vi "Actor Core.vi"(8 "error in":errorcluster, 11 "Monitor in":refnum<class "Classic Monitor.lvclass">) -> (0 "error out":errorcluster, 3 "Actor out":refnum<class "Actor.lvclass">)   [LabVIEW 2023, in "Monitored Actor.lvlib" / "Classic Monitor.lvclass"]
doc: "(<B>Filename</B>: Actor Framework.lvlib:Actor.lvclass:Actor Core.vi)\n\nReceives messages to the actor, reacts to them, and initiates any error handling that may shut the actor down.\n\nDescendant classes may override this VI to append parallel tasks for the actor to complete while it handles messages. Overrides use the Call Parent Method node."
uses:
  Classic Monitor.lvclass
  C:/Users/Public/Documents/Development/builds/Framework/Actor Framework.lvlibp/1abvi3w/vi.lib/ActorFramework/Actor/Actor.lvclass
  builds/Framework/Actor Framework.lvlibp/1abvi3w/vi.lib/ActorFramework/Actor/Actor.lvclass
  Monitor Data/Monitor Data.lvclass
  builds/Framework/Actor Framework.lvlibp/1abvi3w/vi.lib/ActorFramework/Message Enqueuer/Message Enqueuer.lvclass
  Classic Monitor.lvclass/Classic Monitor.ctl
  builds/Framework/Actor Framework.lvlibp/1abvi3w/vi.lib/ActorFramework/Time-Delayed Send Message/Time-Delay Override Options.ctl
  Orphan Detector/Orphan Detector/Orphan Detector.lvclass
  Actor Monitor/Actor Monitor Messages/Ping Actor Msg/Ping Actor Msg.lvclass
  C:/Users/Public/Documents/Development/builds/Framework/Actor Framework.lvlibp/1abvi3w/vi.lib/ActorFramework/Message/Message.lvclass
  Actor Monitor/Actor Monitor/Actor Monitor.lvclass
  Actor Monitor/Actor Monitor Messages/Manually Remove Actor Msg/Manually Remove Actor Msg.lvclass
  Monitor Messages/Log Messages Msg/Log Messages Msg.lvclass
  builds/Framework/Actor Framework.lvlibp/1abvi3w/vi.lib/ActorFramework/Stop Msg/Stop Msg.lvclass
  builds/Framework/Actor Framework.lvlibp
panel:
  in  "Monitored Actors":string[](tree)
  in  "Stop Actor":bool
  in  "Show Actor Core":bool
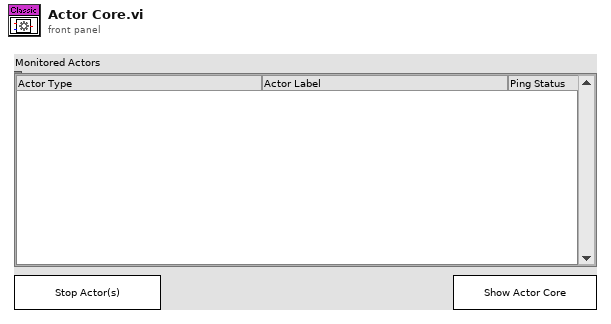
[diagram p1: front panel]
types:
  T1 = enum32{"Invalid", "Standard", "Closed", "Hidden", "Minimized", "Maximized"}
  T2 = cluster{"Monitor Data":refnum<class "Monitor Data.lvclass">, "Changed Actor Q":refnum<class "Message Enqueuer.lvclass">}
  T3 = cluster{"left":i16, "top":i16, "right":i16, "bottom":i16}
  T4 = typedef "Actor Framework.lvlibp/Time-Delay Override Options.ctl" = enum16{"Send next copy now", "Skip next scheduled copy", "Send next copy now and stop all further copies", "Stop all further copies"}
  T5 = enum8{"Enabled", "Disabled", "Disabled and Grayed Out"}
  T6 = typedef "LVRectTypeDef.ctl" = cluster{"Left":i16, "Top":i16, "Right":i16, "Bottom":i16}
  T7 = typedef "LVPoint32TypeDef.ctl" = cluster{"Horizontal":i32, "Vertical":i32}
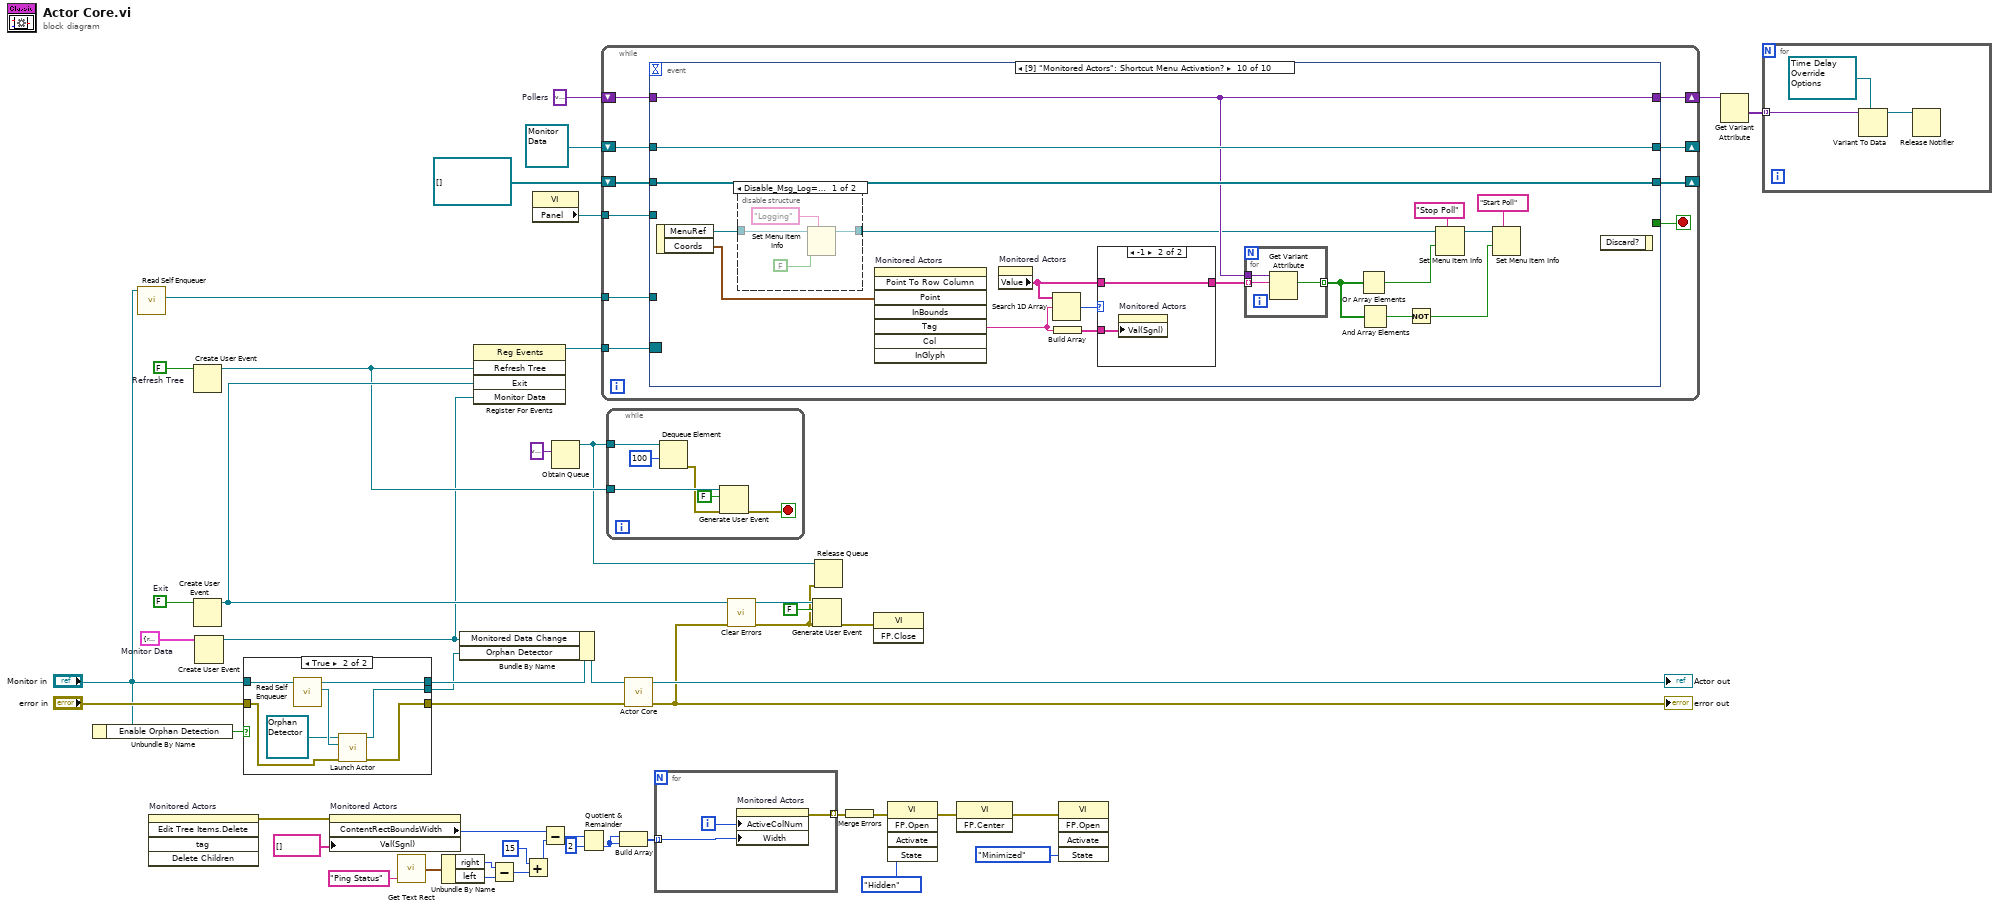
[diagram p0: block diagram]
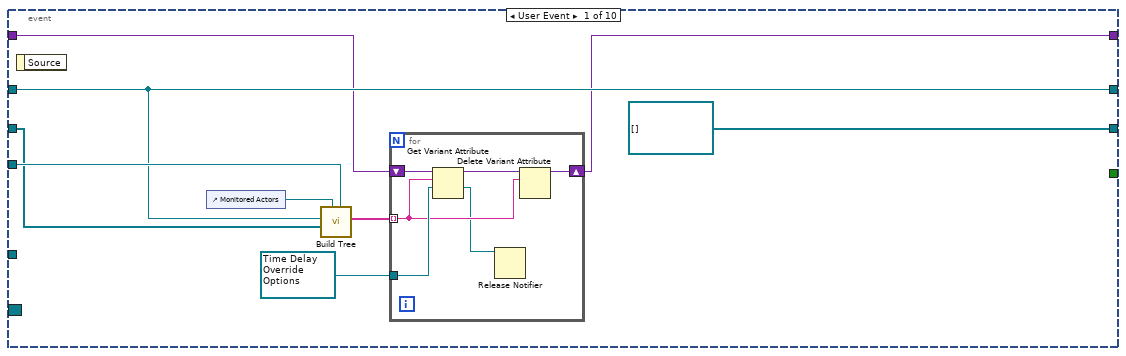
[diagram p3: hidden frame]
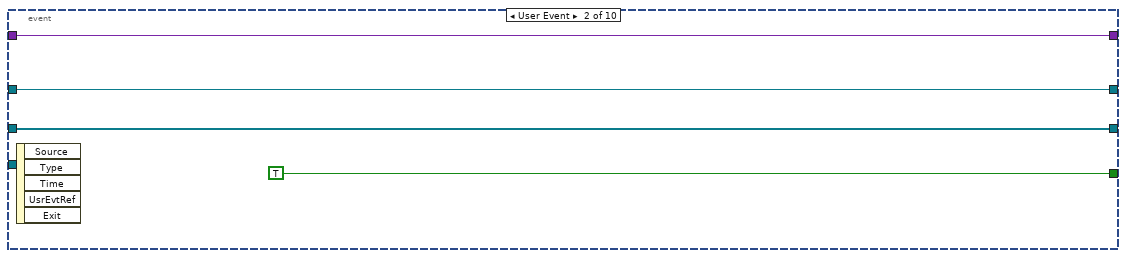
[diagram p4: hidden frame]
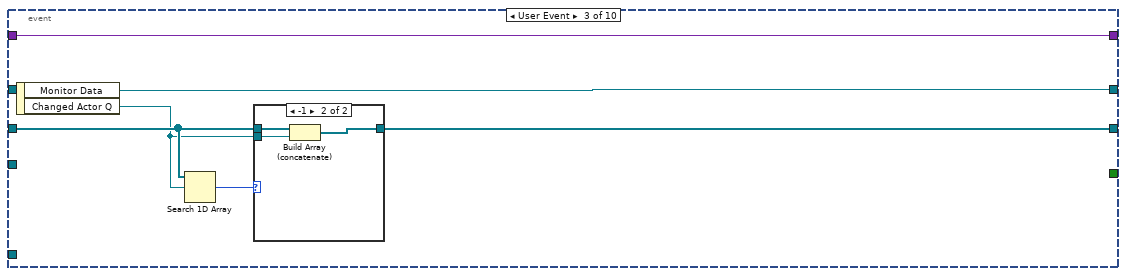
[diagram p5: hidden frame]
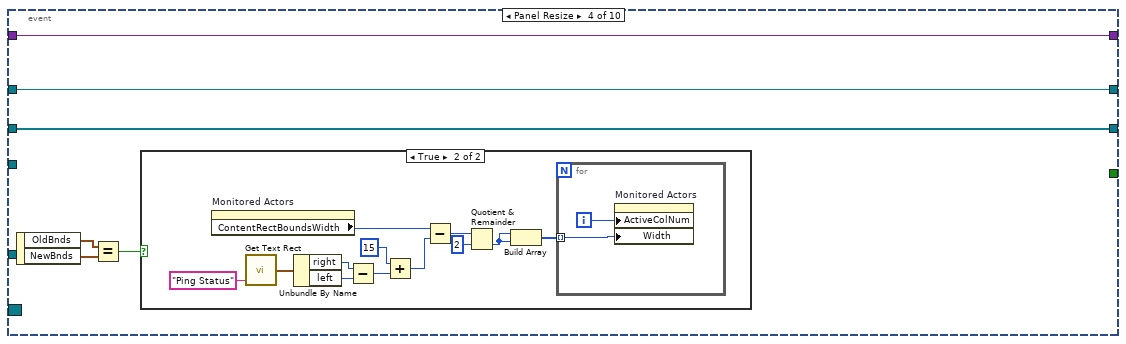
[diagram p7: hidden frame]
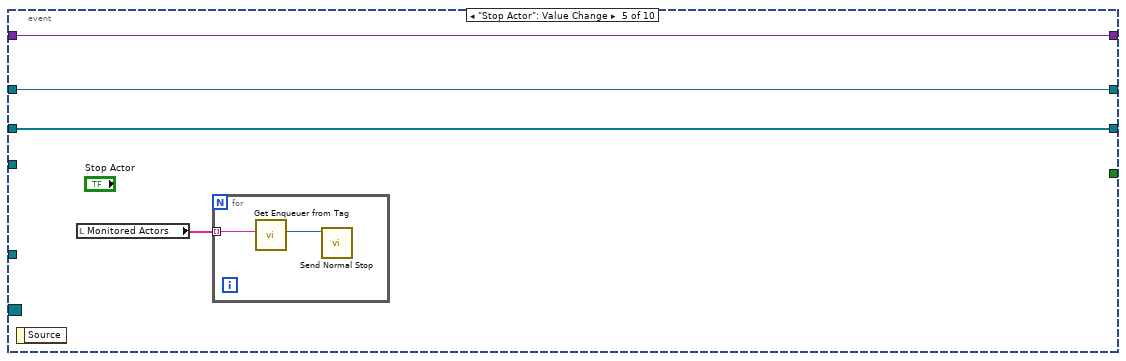
[diagram p9: hidden frame]
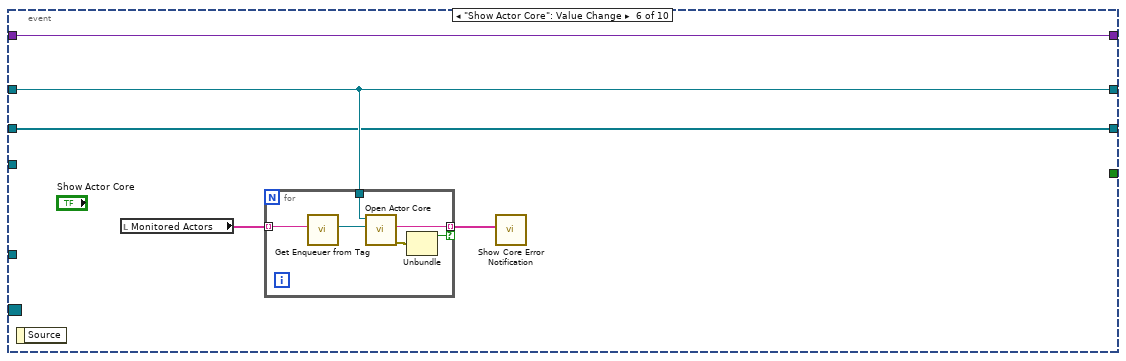
[diagram p10: hidden frame]
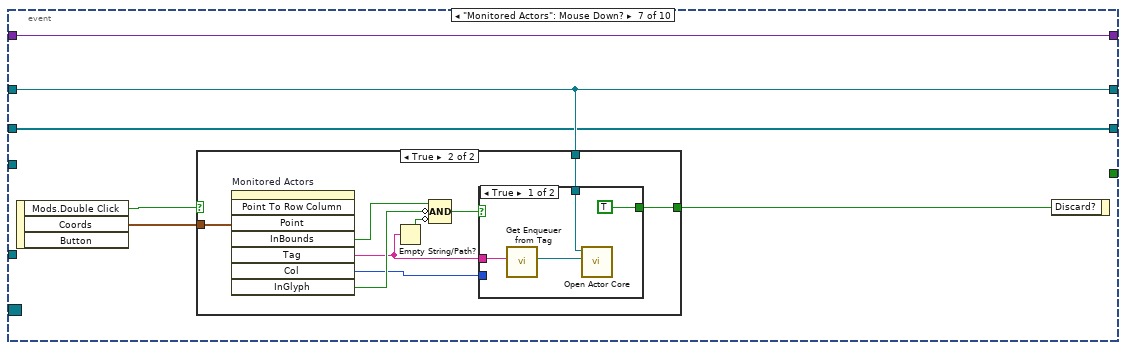
[diagram p11: hidden frame]
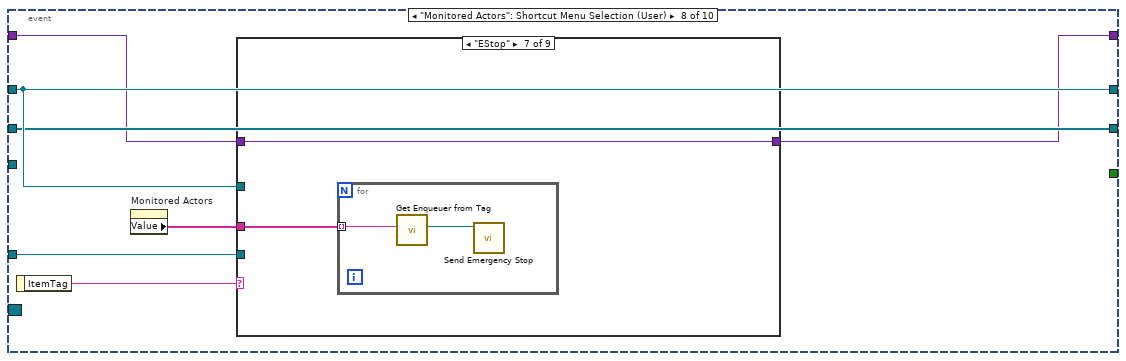
[diagram p14: hidden frame]
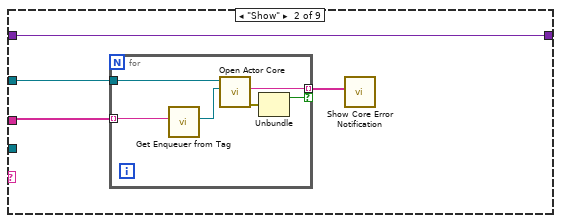
[diagram p16: hidden frame]
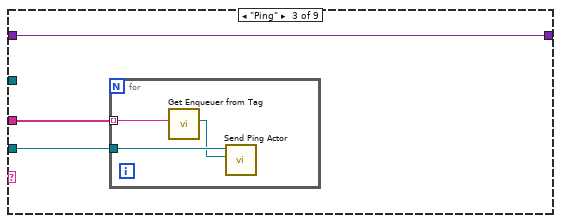
[diagram p17: hidden frame]
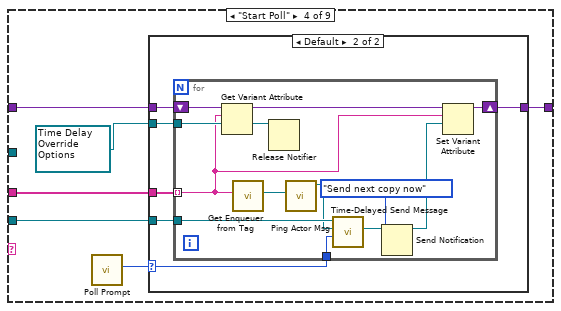
[diagram p18: hidden frame]
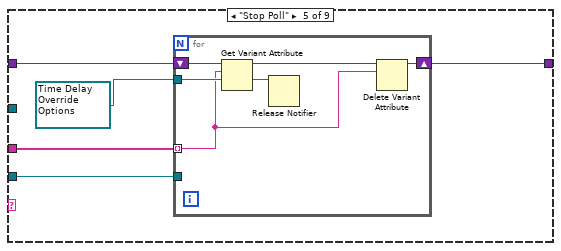
[diagram p20: hidden frame]
diagram:
  w5 = variant  # Pollers
  w15 = T2 {"Monitor Data"=refnum, "Changed Actor Q"=refnum}  # Monitor Data
  w20 = FALSE  # Refresh Tree
  w33 = FALSE  # Exit
  n1 = Unbundle By Name("Monitor in") -> ("Enable Orphan Detection"=w6:bool)
  n2 = call "Read Self Enqueuer.vi"("Actor"="Monitor in") -> ("Self Enqueuer"=w27:refnum<class "Message Enqueuer.lvclass">)  [unwired: 10 in]
  n3 = invoke on="Monitored Actors" class="Tree (strict)" method="Edit Tree Items.Delete"() -> (error out=w12:errorcluster)  [unwired: 5 in, 4 out]
  n4 = Create User Event(user event datatype=w20) -> (user event=w19:refnum<user-event>)  [unwired: 1 in, 1 out]
  n5 = Create User Event(user event datatype=w33) -> (user event=w32:refnum<user-event>)  [unwired: 1 in, 1 out]
  n6 = Create User Event(user event datatype=w15) -> (user event=w14:refnum<user-event>)  [unwired: 1 in, 1 out]
  n7 = case shown="True" w6 {
    tunnel: "error in" -> [w49 w52]
    tunnel: [w49 w51] -> w11
    tunnel: [w50 w55] -> w10
    tunnel: "Monitor in" -> [w50 w55]
    tunnel: [_ w53] -> w9
    frame False {
    }
    frame True {
      n8 = call "Read Self Enqueuer.vi"("Actor"=w55) -> ("Self Enqueuer"=w56:refnum<class "Message Enqueuer.lvclass">)  [unwired: 10 in]
      n9 = call "Launch Actor.vi"("error in (no error)"=w52, "Actor-to-Caller Enqueuer"=w56, "Actor"=refnum<class "Orphan Detector.lvclass"> refnum ("Classic Monitor.lvlib:Orphan Detector.lvclass")) -> ("error out"=w51:errorcluster, "Caller-To-Actor Enqueuer"=w53:refnum<class "Message Enqueuer.lvclass">)  [unwired: 7 in]
    }
  }
  n10 = property on="Monitored Actors" class="Tree (strict)"(error in=w12, "Val(Sgnl)"=string[] [] ("Value (Signaling)")) -> ("ContentRectBoundsWidth"=w46:i32)  [unwired: 1 in, 2 out]
  n11 = call <vilib>:"Get Text Rect.vi"("text"="Ping Status") -> ("rect"=w44:T3)  [unwired: 8 in]
  n12 = Unbundle By Name(w44) -> ("right"=w43:i16, "left"=w42:i16)
  n13 = Bundle By Name(cluster=w10, "Monitored Data Change"=w14, "Orphan Detector"=w9) -> (w30:refnum<class "Classic Monitor.lvclass">)
  n14 = register-events(w19, w32, w14) -> (reference out=w34:refnum<event-registration>)  [unwired: 2 in, 1 out]
  n15 = Subtract(x=w43, y=w42) -> (x-y=w41:i16)
  n16 = Add(x=i16 15, y=w41) -> (x+y=w38:i16)
  n17 = property class="VI"() -> ("Panel"=w28:refnum<vi>)  [unwired: 2 in, 2 out]
  n18 = Subtract(x=w46, y=w38) -> (x-y=w40:i32)
  n19 = Obtain Queue(element data type=variant) -> (queue out=w16:refnum<queue>)  [unwired: 4 in, 2 out]
  n20 = Quotient & Remainder(x=w40, y=2) -> (floor(x/y)=w36:i32)  [unwired: 1 out]
  n21 = while {
    tunnel: w34 -> [w66]
    shift-right: [w64] -> _
    shift-left: refnum<class "Monitor Data.lvclass"> refnum ("Monitor Data") -> [w63]
    tunnel: w28 -> [w62]
    tunnel: w27 -> [w61]
    shift-right: [w60] -> _
    shift-left: refnum<class "Message Enqueuer.lvclass">[] [] -> [w59]
    shift-right: [w58] -> w4
    shift-left: w5 -> [w57]
    stop <- w65 stop-if-true
    n22 = event shown="[9] \"Monitored Actors\": Shortcut Menu Activation?" {
      selector: w66 -> [_ _ _ _ _ _ _ _ _ _]
      dyn-events: _ -> [_ _ _ _ _ _ _ _ _ _]
      timeout: _ -> [_ _ _ _ _ _ _ _ _ _]
      tunnel: [_ TRUE _ _ _ _ _ _ _ _] -> w65
      tunnel: [w74 w84 w91 w101 w119 w125 w138 w158 w243 w260] -> w64
      tunnel: w63 -> [w74 w84 _ w101 w119 w125 w138 w158 w243 w260]
      tunnel: w62 -> [w75 _ _ _ _ _ _ _ _ _]
      tunnel: w61 -> [_ _ _ _ _ _ _ w155 _ _]
      tunnel: [refnum<class "Message Enqueuer.lvclass">[] [] w83 w90 w97 w117 w124 w134 w154 w244 w262] -> w60
      tunnel: w59 -> [w72 w83 w89 w97 w117 w124 w134 w154 w244 w262]
      tunnel: [w67 w82 w86 w96 w116 w122 w133 w152 w237 w253] -> w58
      tunnel: w57 -> [w68 w82 w86 w96 w116 w122 w133 w153 w237 w253]
      event User Event {
        w69 = refnum<notifier> refnum items=["Send next copy now", "Skip next scheduled copy", "Send next copy now and stop all further copies", "Stop all further copies"] ("Delivery Notifier")
        n23 = event-data() -> ()  [unwired: 1 in, 1 out]
        n24 = control-ref of="Monitored Actors"() -> (w73:refnum<vi>)
        n25 = call "Build Tree.vi"("Panel"=w75, "Tree"=w73, "Changed Actors"=w72, "Monitor Data"=w74) -> ("Stopped Actors"=w70:string[])  [unwired: 7 in]
        n26 = for {
          tunnel: w70 -> [w78] mode=indexing
          shift-right: [w77] -> w67
          shift-left: w68 -> [w81]
          tunnel: w69 -> [w80]
          n27 = Get Variant Attribute(Variant=w81, name=w78, default value (empty Variant)=w80) -> (duplicate Variant=w79:variant, value=w76:refnum<notifier>)  [unwired: 1 in, 2 out]
          n28 = Release Notifier(notifier=w76) -> ()  [unwired: 2 in, 3 out]
          n29 = Delete Variant Attribute(6:w78, 7:w79) -> (3:w77:variant)  [unwired: 1 in, 2 out]
        }
      }
      event User Event {
        n30 = event-data() -> ()  [unwired: 1 in, 5 out]
      }
      event User Event {
        n31 = event-data() -> ("Monitor Data"=w91:refnum<class "Monitor Data.lvclass">, "Changed Actor Q"=w88:refnum<class "Message Enqueuer.lvclass">)  [unwired: 1 in]
        n32 = Search 1D Array(1D array=w89, element=w88) -> (index of element=w87:i32)  [unwired: 1 in]
        n33 = case shown="-1" w87 {
          tunnel: [w92 w95] -> w90
          tunnel: w89 -> [w92 w94]
          tunnel: w88 -> [_ w93]
          frame Default {
          }
          frame -1 {
            n34 = Build Array (concatenate)(w94, w93) -> (w95:refnum<class "Message Enqueuer.lvclass">[])
          }
        }
      }
      event Panel Resize {
        n35 = event-data() -> ("OldBnds"=w100:T6, "NewBnds"=w99:T6)  [unwired: 1 in]
        n36 = Equal?(x=w100, y=w99) -> (x = y?=w98:bool)
        n37 = case shown="True" w98 {
          frame False {
          }
          frame True {
            n38 = property on="Monitored Actors" class="Tree (strict)"() -> ("ContentRectBoundsWidth"=w102:i32)  [unwired: 2 in, 2 out]
            n39 = call <vilib>:"Get Text Rect.vi"("text"="Ping Status") -> ("rect"=w104:T3)  [unwired: 8 in]
            n40 = Unbundle By Name(w104) -> ("right"=w105:i16, "left"=w106:i16)
            n41 = Subtract(x=w105, y=w106) -> (x-y=w107:i16)
            n42 = Add(x=i16 15, y=w107) -> (x+y=w110:i16)
            n43 = Subtract(x=w102, y=w110) -> (x-y=w108:i32)
            n44 = Quotient & Remainder(x=w108, y=2) -> (floor(x/y)=w112:i32)  [unwired: 1 out]
            n45 = Build Array(w112, w112) -> (w113:i32[])
            n46 = for {
              tunnel: w113 -> [w114] mode=indexing
              i -> [w115]
              n47 = property on="Monitored Actors" class="Tree (strict)"("ActiveColNum"=w115, "Width"=w114) -> ()  [unwired: 2 in, 2 out]
            }
          }
        }
      }
      event "Stop Actor": Value Change {
        n48 = event-data() -> ()  [unwired: 1 in, 1 out]
        n49 = local read "Monitored Actors"() -> (w118:string[])
        n50 = for {
          tunnel: w118 -> [w121] mode=indexing
          n51 = call "Get Enqueuer from Tag.vi"("Tag"=w121) -> ("Enqueuer"=w120:refnum<class "Message Enqueuer.lvclass">)  [unwired: 10 in]
          n52 = call "Send Normal Stop.vi"("Message Enqueuer"=w120) -> ()  [unwired: 10 in, 1 out]
        }
      }
      event "Show Actor Core": Value Change {
        n53 = event-data() -> ()  [unwired: 1 in, 1 out]
        n54 = local read "Monitored Actors"() -> (w126:string[])
        n55 = for {
          tunnel: w126 -> [w132] mode=indexing
          tunnel: w125 -> [w131]
          tunnel: [w129] -> w123 mode=indexing if=w127
          n56 = call "Get Enqueuer from Tag.vi"("Tag"=w132) -> ("Enqueuer"=w130:refnum<class "Message Enqueuer.lvclass">)  [unwired: 10 in]
          n57 = call "Open Actor Core.vi"("Actor's Self Q"=w130, "Monitor Data"=w131) -> ("error out"=w128:errorcluster, "Actor Core VI"=w129:string)  [unwired: 8 in]
          n58 = Unbundle(w128) -> ("status"=w127:bool)  [unwired: 2 out]
        }
        n59 = call "Show Core Error Notification.vi"("Error VIs"=w123) -> ()  [unwired: 11 in]
      }
      event "Monitored Actors": Mouse Down? {
        n60 = event-data() -> ("Mods.Double Click"=w137:bool, "Coords"=w136:T7)  [unwired: 1 in, 1 out]
        n61 = case shown="True" w137 {
          tunnel: w138 -> [_ w147]
          tunnel: w136 -> [_ w146]
          tunnel: [_ w143] -> w135
          frame False {
          }
          frame True {
            n62 = invoke on="Monitored Actors" class="Tree (strict)" method="Point To Row Column"("Point"=w146) -> ("InBounds"=w145:bool, "Tag"=w140:string, "Col"=w139:i32, "InGlyph"=w144:bool)  [unwired: 7 in, 4 out]
            n63 = Empty String/Path?(string/path=w140) -> (empty?=w141:bool)
            n64 = Compound Arithmetic op=AND(w145, invert w144, invert w141) -> (w142:bool)
            n65 = case shown="True" w142 {
              tunnel: w147 -> [w149 _]
              tunnel: [TRUE _] -> w143
              tunnel: w140 -> [w151 _]
              tunnel: w139 -> [_ _]
              frame True {
                n66 = call "Get Enqueuer from Tag.vi"("Tag"=w151) -> ("Enqueuer"=w148:refnum<class "Message Enqueuer.lvclass">)  [unwired: 10 in]
                n67 = call "Open Actor Core.vi"("Actor's Self Q"=w148, "Monitor Data"=w149) -> ()  [unwired: 8 in, 2 out]
              }
              frame False {
              }
            }
          }
        }
        n68 = event-data("Discard?"=w135) -> ()  [unwired: 1 in, 1 out]
      }
      event "Monitored Actors": Shortcut Menu Selection (User) {
        n69 = event-data() -> ("ItemTag"=w157:string)  [unwired: 1 in]
        n70 = property on="Monitored Actors" class="Tree (strict)"() -> ("Value"=w156:string[])  [unwired: 2 in, 2 out]
        n71 = case shown="\"EStop\"" w157 {
          tunnel: w158 -> [_ w162 _ _ _ _ _ _ _]
          tunnel: w156 -> [_ w163 w172 w181 w206 w214 w218 w225 w233]
          tunnel: w155 -> [_ _ w171 w180 w205 _ _ w224 w232]
          tunnel: w153 -> [w159 w160 w170 w179 w204 w213 w217 w223 w231]
          tunnel: [w159 w160 w170 w178 w203 w213 w217 w223 w231] -> w152
          frame Default {
          }
          frame "Show" {
            n72 = for {
              tunnel: w163 -> [w169] mode=indexing
              tunnel: w162 -> [w168]
              tunnel: [w166] -> w161 mode=indexing if=w164
              n73 = call "Get Enqueuer from Tag.vi"("Tag"=w169) -> ("Enqueuer"=w167:refnum<class "Message Enqueuer.lvclass">)  [unwired: 10 in]
              n74 = call "Open Actor Core.vi"("Actor's Self Q"=w167, "Monitor Data"=w168) -> ("error out"=w165:errorcluster, "Actor Core VI"=w166:string)  [unwired: 8 in]
              n75 = Unbundle(w165) -> ("status"=w164:bool)  [unwired: 2 out]
            }
            n76 = call "Show Core Error Notification.vi"("Error VIs"=w161) -> ()  [unwired: 11 in]
          }
          frame "Ping" {
            n77 = for {
              tunnel: w172 -> [w175] mode=indexing
              tunnel: w171 -> [w174]
              n78 = call "Get Enqueuer from Tag.vi"("Tag"=w175) -> ("Enqueuer"=w173:refnum<class "Message Enqueuer.lvclass">)  [unwired: 10 in]
              n79 = call "Send Ping Actor.vi"("Actor"=w173, "Message Enqueuer in"=w174) -> ()  [unwired: 8 in, 2 out]
            }
          }
          frame "Start Poll" {
            w177 = refnum<notifier> refnum items=["Send next copy now", "Skip next scheduled copy", "Send next copy now and stop all further copies", "Stop all further copies"] ("Delivery Notifier")
            n80 = call "Poll Prompt.vi"() -> ("Period"=w176:i32)  [unwired: 10 in, 1 out]
            n81 = case shown="Default" w176 {
              selector: w176 -> [_ w183]
              tunnel: w181 -> [_ w188]
              tunnel: w180 -> [_ w187]
              tunnel: w179 -> [w182 w186]
              tunnel: [w182 w185] -> w178
              tunnel: w177 -> [_ w184]
              frame -1 {
              }
              frame Default {
                n82 = for {
                  tunnel: w188 -> [w192] mode=indexing
                  tunnel: w187 -> [w201]
                  shift-right: [w194] -> w185
                  shift-left: w186 -> [w198]
                  tunnel: w184 -> [w196]
                  tunnel: w183 -> [w191]
                  n83 = Get Variant Attribute(Variant=w198, name=w192, default value (empty Variant)=w196) -> (duplicate Variant=w197:variant, value=w195:refnum<notifier>)  [unwired: 1 in, 2 out]
                  n84 = call "Get Enqueuer from Tag.vi"("Tag"=w192) -> ("Enqueuer"=w200:refnum<class "Message Enqueuer.lvclass">)  [unwired: 10 in]
                  n85 = Release Notifier(notifier=w195) -> ()  [unwired: 2 in, 3 out]
                  n86 = call "Ping Actor Msg.vi"("Actor"=w200) -> ("Ping Actor Msg out"=w199:refnum<class "Ping Actor Msg.lvclass">)  [unwired: 9 in, 1 out]
                  n87 = call "Time-Delayed Send Message.vi"("Milliseconds To Wait"=w191, "Message"=w199, "Message Enqueuer"=w201) -> ("Delivery Notifier"=w193:refnum<notifier>)  [unwired: 7 in, 1 out]
                  n88 = Send Notification(notification=Time-Delay_Override_Options."Send next copy now" ("Time Delay Override Options"), notifier=w193) -> (notifier out=w190:refnum<notifier>)  [unwired: 1 in, 1 out]
                  n89 = Set Variant Attribute(Variant=w197, name=w192, value=w190) -> (Variant out=w194:variant)  [unwired: 1 in, 2 out]
                }
              }
            }
          }
          frame "Stop Poll" {
            w202 = refnum<notifier> refnum items=["Send next copy now", "Skip next scheduled copy", "Send next copy now and stop all further copies", "Stop all further copies"] ("Delivery Notifier")
            n90 = for {
              tunnel: w206 -> [w207] mode=indexing
              tunnel: w205 -> [_]
              shift-right: [w208] -> w203
              shift-left: w204 -> [w212]
              tunnel: w202 -> [w210]
              n91 = Get Variant Attribute(Variant=w212, name=w207, default value (empty Variant)=w210) -> (duplicate Variant=w211:variant, value=w209:refnum<notifier>)  [unwired: 1 in, 2 out]
              n92 = Release Notifier(notifier=w209) -> ()  [unwired: 2 in, 3 out]
              n93 = Delete Variant Attribute(6:w207, 7:w211) -> (3:w208:variant)  [unwired: 1 in, 2 out]
            }
          }
          frame "Stop" {
            n94 = for {
              tunnel: w214 -> [w216] mode=indexing
              n95 = call "Get Enqueuer from Tag.vi"("Tag"=w216) -> ("Enqueuer"=w215:refnum<class "Message Enqueuer.lvclass">)  [unwired: 10 in]
              n96 = call "Send Normal Stop.vi"("Message Enqueuer"=w215) -> ()  [unwired: 10 in, 1 out]
            }
          }
          frame "EStop" {
            n97 = for {
              tunnel: w218 -> [w220] mode=indexing
              n98 = call "Get Enqueuer from Tag.vi"("Tag"=w220) -> ("Enqueuer"=w219:refnum<class "Message Enqueuer.lvclass">)  [unwired: 10 in]
              n99 = call "Send Emergency Stop.vi"("Message Enqueuer"=w219) -> ()  [unwired: 10 in, 1 out]
            }
          }
          frame "Remove" {
            n100 = Two Button Dialog(message="Warning: Manually removing actors from list can lead to inconsitancies between the monitor and the actual state.\n\n Only do this if you're sure the actor has been aborted manually.") -> (T button?=w221:bool)  [unwired: 2 in]
            n101 = case shown="True" w221 {
              tunnel: w225 -> [_ w227]
              tunnel: w224 -> [_ w226]
              frame False {
              }
              frame True {
                n102 = for {
                  tunnel: w227 -> [w230] mode=indexing
                  tunnel: w226 -> [w228]
                  n103 = call "Get Enqueuer from Tag.vi"("Tag"=w230) -> ("Enqueuer"=w229:refnum<class "Message Enqueuer.lvclass">)  [unwired: 10 in]
                  n104 = call "Send Manually Remove Actor.vi"("Actor's Q"=w229, "Message Enqueuer in"=w228) -> ()  [unwired: 8 in, 2 out]
                }
              }
            }
          }
          frame "Logging" {
            n105 = for {
              tunnel: w233 -> [w236] mode=indexing
              tunnel: w232 -> [w235]
              n106 = call "Get Enqueuer from Tag.vi"("Tag"=w236) -> ("Enqueuer"=w234:refnum<class "Message Enqueuer.lvclass">)  [unwired: 10 in]
              n107 = call "Send Log Messages.vi"("Actor to Log"=w234, "Message Enqueuer in"=w235) -> ()  [unwired: 8 in, 2 out]
            }
          }
        }
      }
      event "Monitored Actors": Value Change {
        n108 = event-data() -> ()  [unwired: 1 in, 1 out]
        n109 = Empty Array?(array="Monitored Actors") -> (empty?=w241:bool)
        n110 = Select(t=T5."Disabled and Grayed Out" ("Disabled"), s=w241, f=T5."Enabled") -> (s? t:f=w238:T5)
        n111 = property on="Stop Actor" class="Bool"("DisabledEnum"=w238) -> ()  [unwired: 2 in, 2 out]
        n112 = property on="Show Actor Core" class="Bool"("DisabledEnum"=w238) -> ()  [unwired: 2 in, 2 out]
      }
      event "Monitored Actors": Shortcut Menu Activation? {
        n113 = event-data() -> ("MenuRef"=w261:refnum<k9>, "Coords"=w259:T7)  [unwired: 1 in]
        n114 = disable-structure shown="Disable_Msg_Log==True" {
          disable-tunnel: w261 -> [w272 w273]
          disable-tunnel: [w269 w273] -> w251
          frame condition #0 {
            n115 = Set Menu Item Info(7:"Logging" ("item name"), 9:FALSE ("enabled"), 11:w272) -> (3:w269:refnum<k9>)  [unwired: 4 in, 1 out]
          }
          frame condition #1 (active) {
          }
        }
        n116 = invoke on="Monitored Actors" class="Tree (strict)" method="Point To Row Column"("Point"=w259) -> ("Tag"=w258:string)  [unwired: 7 in, 7 out]
        n117 = property on="Monitored Actors" class="Tree (strict)"() -> ("Value"=w255:string[])  [unwired: 2 in, 2 out]
        n118 = Search 1D Array(1D array=w255, element=w258) -> (index of element=w256:i32)  [unwired: 1 in]
        n119 = Build Array(w258) -> (w257:string[])
        n120 = case shown="-1" w256 {
          tunnel: w257 -> [_ w268]
          tunnel: w255 -> [w266 w267]
          tunnel: [w266 w267] -> w254
          frame Default {
          }
          frame -1 {
            n121 = property on="Monitored Actors" class="Tree (strict)"("Val(Sgnl)"=w268) -> ()  [unwired: 2 in, 2 out]
          }
        }
        n122 = for {
          tunnel: w254 -> [w264] mode=indexing
          tunnel: w253 -> [w265]
          tunnel: [w263] -> w248 mode=indexing
          n123 = Get Variant Attribute(Variant=w265, name=w264) -> (found=w263:bool)  [unwired: 2 in, 3 out]
        }
        n124 = Or Array Elements(Boolean array=w248) -> (logical OR=w245:bool)
        n125 = And Array Elements(Boolean array=w248) -> (logical AND=w247:bool)
        n126 = Not(x=w247) -> (.not. x?=w246:bool)
        n127 = Set Menu Item Info(7:"Stop Poll" ("item name"), 9:w245, 11:w251) -> (3:w250:refnum<k9>)  [unwired: 4 in, 1 out]
        n128 = Set Menu Item Info(7:"Start Poll" ("item tag"), 9:w246, 11:w250) -> ()  [unwired: 4 in, 2 out]
        n129 = event-data() -> ()  [unwired: 2 in, 1 out]
      }
    }
  }
  n130 = while {
    tunnel: w16 -> [w278]
    tunnel: w19 -> [w277]
    stop <- w275 stop-if-true
    n131 = Dequeue Element(queue=w278, timeout in ms (-1)=100) -> (error out=w276:errorcluster)  [unwired: 1 in, 3 out]
    n132 = Generate User Event(user event=w277, event data cluster=FALSE ("event data"), error in=w276) -> (error out=w275:errorcluster)  [unwired: 1 in, 1 out]
  }
  n133 = Build Array(w36, w36) -> (w35:i32[])
  n134 = call-parent "Actor Core.vi"("error in"=w11, "Actor in"=w30) -> ("error out"=w31:errorcluster, "Actor out"=→"Actor out":refnum<class "Actor.lvclass">)  [unwired: 8 in]
  "error out" <- w31
  n135 = for {
    tunnel: w35 -> [w281] mode=indexing
    tunnel: [w280] -> w26 mode=indexing
    i -> [w282]
    n136 = property on="Monitored Actors" class="Tree (strict)"("ActiveColNum"=w282, "Width"=w281) -> (error out=w280:errorcluster)  [unwired: 2 in, 1 out]
  }
  n137 = call <vilib>:"Clear Errors.vi"("error in (no error)"=w31) -> ("error out"=w17:errorcluster)  [unwired: 5 in, 1 out]
  n138 = Generate User Event(user event=w32, event data cluster=FALSE ("event data"), error in=w17) -> (error out=w25:errorcluster)  [unwired: 1 in, 1 out]
  n139 = Release Queue(queue=w16, error in (no error)=w17) -> ()  [unwired: 1 in, 3 out]
  n140 = Merge Errors(w26) -> (w23:errorcluster)
  n141 = invoke class="VI" method="FP.Close"(error in=w25) -> ()  [unwired: 2 in, 3 out]
  n142 = invoke class="VI" method="FP.Open"(error in=w23, "State"=T1."Hidden") -> (error out=w24:errorcluster)  [unwired: 3 in, 4 out]
  n143 = invoke class="VI" method="FP.Center"(error in=w24) -> (error out=w22:errorcluster)  [unwired: 2 in, 2 out]
  n144 = invoke class="VI" method="FP.Open"(error in=w22, "State"=T1."Minimized") -> ()  [unwired: 3 in, 5 out]
  n145 = Get Variant Attribute(Variant=w4) -> (values=w3:variant[])  [unwired: 3 in, 3 out]
  n146 = for {
    tunnel: w3 -> [w285] mode=indexing
    w284 = refnum<notifier> refnum items=["Send next copy now", "Skip next scheduled copy", "Send next copy now and stop all further copies", "Stop all further copies"] ("Delivery Notifier")
    n147 = Variant To Data(type=w284, Variant=w285) -> (data=w283:refnum<notifier>)  [unwired: 1 in, 1 out]
    n148 = Release Notifier(notifier=w283) -> ()  [unwired: 2 in, 3 out]
  }
